vi "Deposition System Automation.vi"() -> ()   [LabVIEW 2018]
uses:
  <vilib>/MakerHub/LINX/Public/Peripherals/Digital/Digital Write 1 Chan.vi
  <vilib>/MakerHub/LINX/Public/Peripherals/Digital/Digital Write N Chans.vi
  <vilib>/MakerHub/LINX/Private/Local IO/LinxDigitalWrite.vi
  <vilib>/MakerHub/LINX/Public/Utilities/Check Channel.vi
  <vilib>/MakerHub/LINX/Public/Utilities/Open Serial.vi
  <vilib>/MakerHub/LINX/Private/Utilties/Generate Error.vi
  <vilib>/MakerHub/LINX/LMH-LINX.lvlib
panel:
  in  "Crashed?":bool
  in  "Arduino COM":refnum<visa-resource-name>="N/A"
  out "Turn On Turbo Pump":bool
  in  "Shut Down":bool
  in  "Turbo Pump":bool
  out "Turn On Pressure Gauge":bool
  in  "Rough Pump":bool
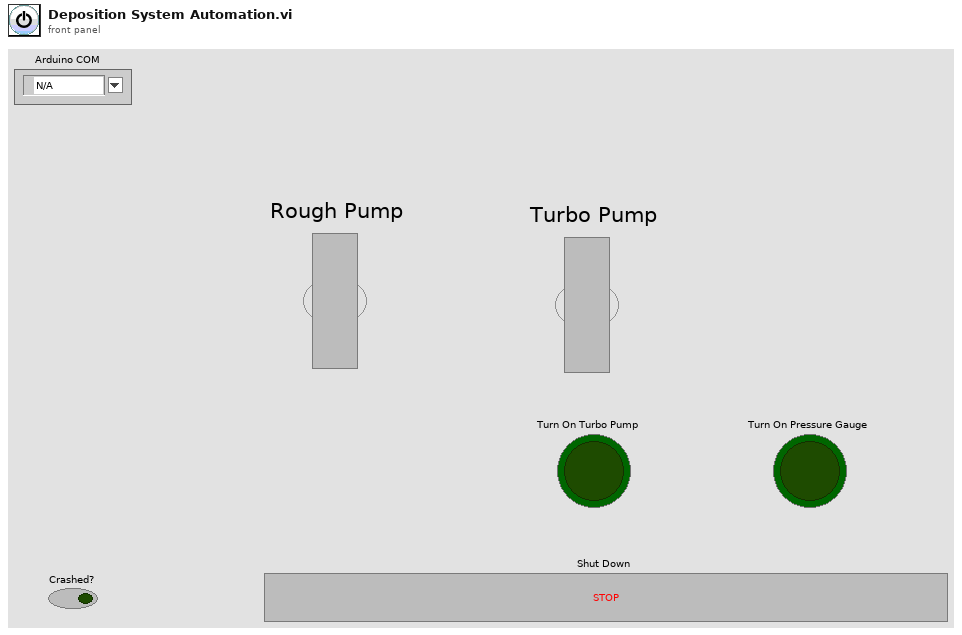
[diagram p1: front panel]
types:
  T1 = typedef "LMH-LINX.lvlib/LINX Ref.ctl" = cluster{"IO":T2, "Interface":T3, "LINX Device Config":T4}
  T2 = typedef "LMH-LINX.lvlib/Platform.ctl" = enum16{"Remote", "Local"}
  T3 = typedef "LMH-LINX.lvlib/Interface.ctl" = enum16{"Serial", "TCP"}
  T4 = typedef "LMH-LINX.lvlib/Device.lvlib/LINX Device Config.ctl" = cluster{"Interface":T3, "COM Port":refnum<visa-resource-name>, "TCP Configuration":T5, "Device Family":u8, "Device ID":u8, "Device Name":string, "TCP Ref":refnum<k5>, "Channels":T6}
  T5 = typedef "LMH-LINX.lvlib/Device.lvlib/TCP Config.ctl" = cluster{"IP Address":string, "Port":u16}
  T6 = typedef "LMH-LINX.lvlib/Channels.ctl" = cluster{"DI":u8[], "DO":u8[], "AI":u8[], "AO":u8[], "PWM":u8[], "QE":u8[], "UART":u8[], "I2C 2":u8[], "SPI":u8[], "CAN":u8[], "Servo":u8[], "AI Ref (V)":dbl, "AI Resolution (Bits)":u8, "AO Ref (V)":dbl, "AO Resolution (Bits)":u8}
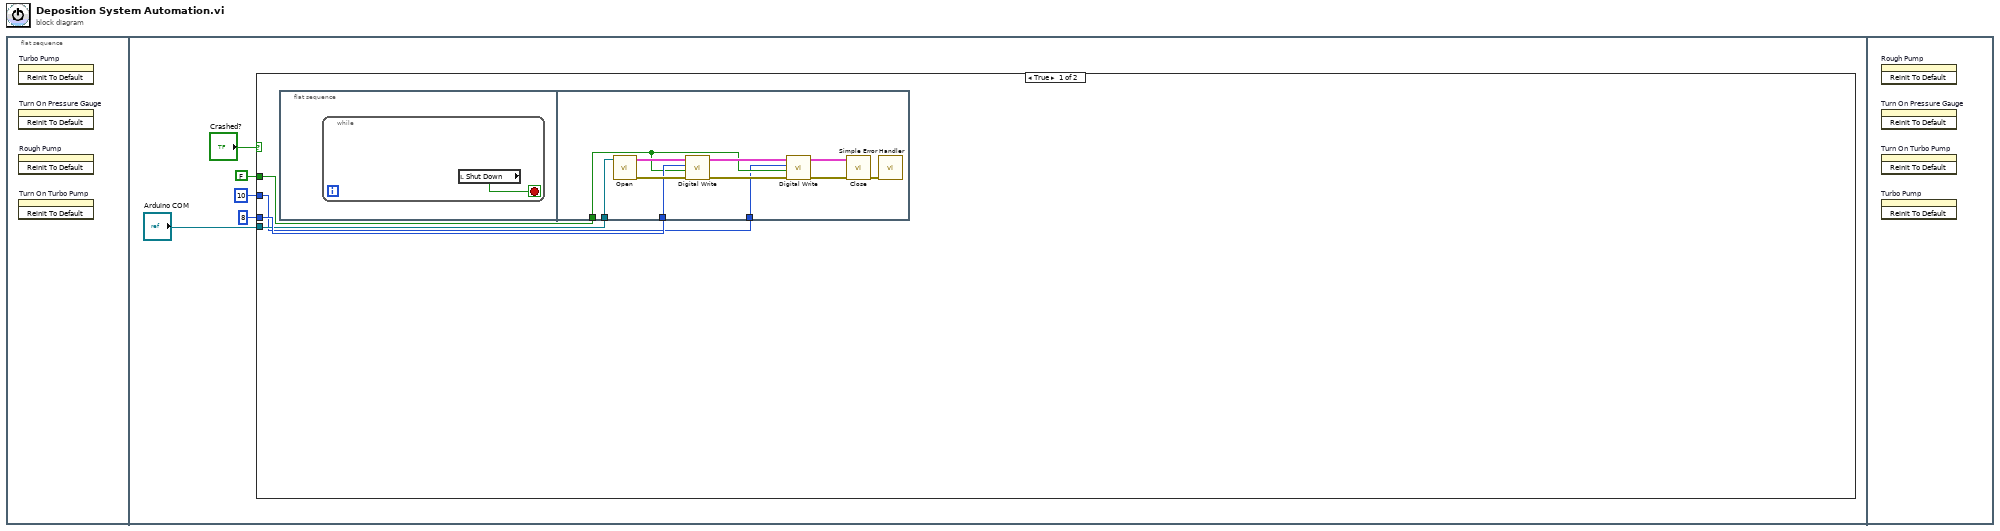
[diagram p0: block diagram]
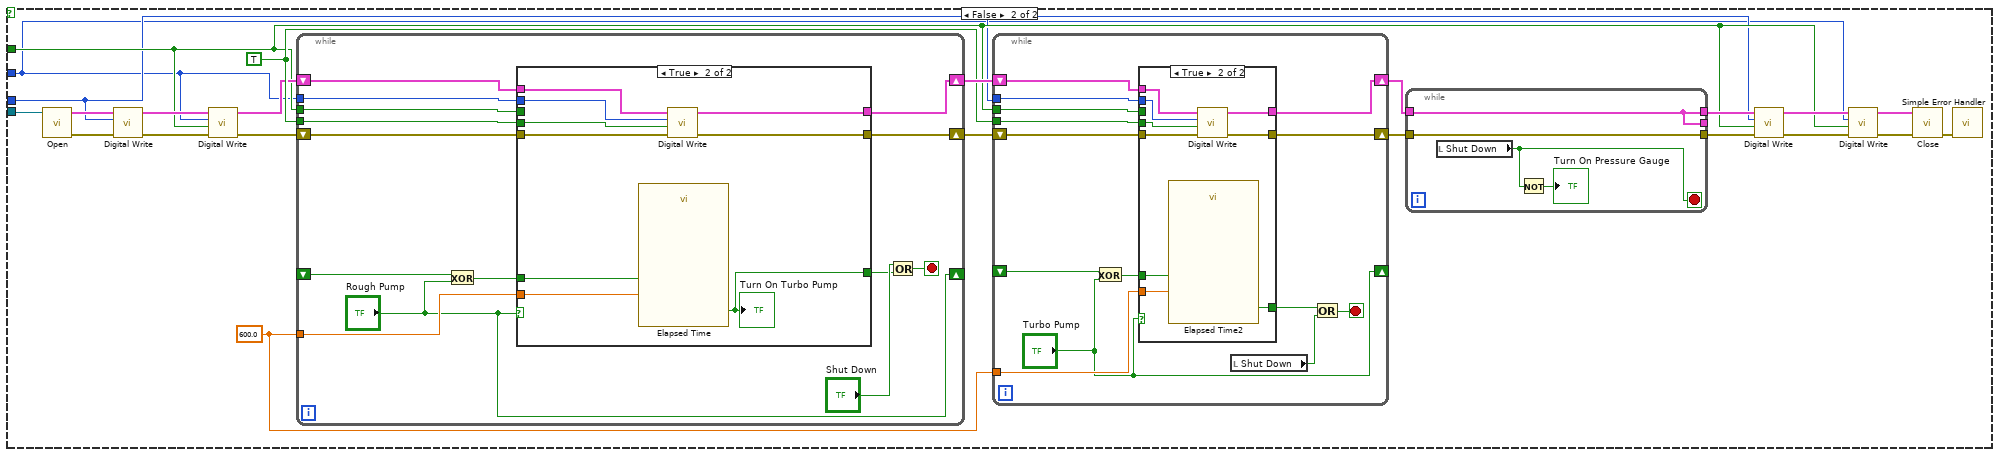
[diagram p2: hidden frame]
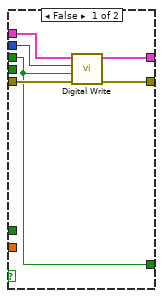
[diagram p3: hidden frame]
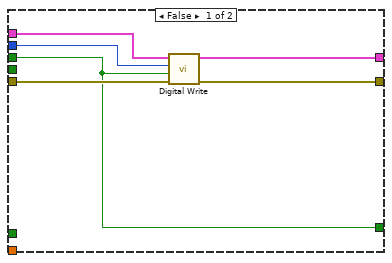
[diagram p4: hidden frame]
diagram:
  n1 = flat-sequence {
    frame #0 {
      n2 = invoke on="Turbo Pump" class="Bool (strict)" method="Reinit To Default"() -> ()  [unwired: 3 in, 3 out]
      n3 = invoke on="Turn On Pressure Gauge" class="Bool (strict)" method="Reinit To Default"() -> ()  [unwired: 3 in, 3 out]
      n4 = invoke on="Rough Pump" class="Bool (strict)" method="Reinit To Default"() -> ()  [unwired: 3 in, 3 out]
      n5 = invoke on="Turn On Turbo Pump" class="Bool (strict)" method="Reinit To Default"() -> ()  [unwired: 3 in, 3 out]
    }
    frame #1 {
      n6 = case shown="True" "Crashed?" {
        tunnel: u8 10 ("DO Channel") -> [w6 w22]
        tunnel: "Arduino COM" -> [w7 w36]
        tunnel: FALSE ("Time has Elapsed") -> [w9 w24]
        tunnel: u8 8 ("DO Channel") -> [w8 w23]
        frame True {
          n7 = flat-sequence {
            tunnel: w9 -> [w12]
            tunnel: w8 -> [w17]
            tunnel: w7 -> [w13]
            tunnel: w6 -> [w11]
            frame #0 {
              n8 = while {
                stop <- w10 stop-if-true
                n9 = local read "Shut Down"() -> (w10:bool)
              }
            }
            frame #1 {
              n10 = call-poly <vilib>:"Open.vi"("Serial Port"=w13) -> ("Error Out"=w19:errorcluster, "LINX Resource"=w18:T1)  [unwired: 8 in, 1 out]
              n11 = call-poly <vilib>:"Digital Write.vi"("Error In"=w19, "Output Value"=w12, "DO Channel"=w17, "LINX Resource"=w18) -> ("Error Out"=w21:errorcluster, "LINX Resource"=w20:T1)  [unwired: 6 in]
              n12 = call-poly <vilib>:"Digital Write.vi"("Error In"=w21, "Output Value"=w12, "DO Channel"=w11, "LINX Resource"=w20) -> ("Error Out"=w14:errorcluster, "LINX Resource"=w15:T1)  [unwired: 6 in]
              n13 = call <vilib>:"Close.vi"("Error In"=w14, "LINX Resource"=w15) -> ("Error Out"=w16:errorcluster)  [unwired: 9 in]
              n14 = call <vilib>:"Simple Error Handler.vi"("error in (no error)"=w16) -> ()  [unwired: 4 in, 5 out]
            }
          }
        }
        frame False {
          w41 = TRUE ("Output Value")
          w42 = 600.0 ("Time Target (s)")
          n15 = call-poly <vilib>:"Open.vi"("Serial Port"=w36) -> ("Error Out"=w35:errorcluster, "LINX Resource"=w34:T1)  [unwired: 8 in, 1 out]
          n16 = call-poly <vilib>:"Digital Write.vi"("Error In"=w35, "DO Channel"=w23, "LINX Resource"=w34) -> ("Error Out"=w40:errorcluster, "LINX Resource"=w39:T1)  [unwired: 7 in]
          n17 = call-poly <vilib>:"Digital Write.vi"("Error In"=w40, "Output Value"=w24, "DO Channel"=w22, "LINX Resource"=w39) -> ("Error Out"=w37:errorcluster, "LINX Resource"=w38:T1)  [unwired: 6 in]
          n18 = while {
            shift-right: [w89] -> w44
            shift-left: w38 -> [w91]
            shift-right: [w88] -> w43
            shift-left: w37 -> [w90]
            tunnel: w42 -> [w87]
            tunnel: w41 -> [w84]
            shift-right: ["Rough Pump"] -> _
            shift-left: _ -> [w82]
            tunnel: w22 -> [w79]
            tunnel: w24 -> [w78]
            stop <- w86 stop-if-true
            n19 = Exclusive Or(1:"Rough Pump", 2:w82) -> (0:w80:bool)
            n20 = case shown="True" "Rough Pump" {
              tunnel: w91 -> [w96 w106]
              tunnel: w90 -> [w95 w105]
              tunnel: w79 -> [w97 w104]
              tunnel: [w94 w103] -> w89
              tunnel: [w93 w102] -> w88
              tunnel: w87 -> [_ w101]
              tunnel: w84 -> [_ w100]
              tunnel: w78 -> [w92 _]
              tunnel: [w92 w99] -> w83
              tunnel: w80 -> [_ w98]
              frame False {
                n21 = call-poly <vilib>:"Digital Write.vi"("Error In"=w95, "Output Value"=w92, "DO Channel"=w97, "LINX Resource"=w96) -> ("Error Out"=w93:errorcluster, "LINX Resource"=w94:T1)  [unwired: 6 in]
              }
              frame True {
                n22 = call "Elapsed Time"("Time Target (s)"=w101, "Reset"=w98) -> ("Time has Elapsed"=w99:bool)  [unwired: 10 in, 7 out]
                "Turn On Turbo Pump" <- w99
                n23 = call-poly <vilib>:"Digital Write.vi"("Error In"=w105, "Output Value"=w100, "DO Channel"=w104, "LINX Resource"=w106) -> ("Error Out"=w102:errorcluster, "LINX Resource"=w103:T1)  [unwired: 6 in]
              }
            }
            n24 = Or(x="Shut Down", y=w83) -> (x .or. y?=w86:bool)
          }
          n25 = while {
            tunnel: w42 -> [w58]
            shift-right: [w62] -> w33
            shift-left: w44 -> [w60]
            shift-right: [w61] -> w32
            shift-left: w43 -> [w59]
            tunnel: w41 -> [w56]
            shift-right: ["Turbo Pump"] -> _
            shift-left: _ -> [w53]
            tunnel: w23 -> [w50]
            tunnel: w24 -> [w49]
            stop <- w54 stop-if-true
            n26 = Exclusive Or(1:"Turbo Pump", 2:w53) -> (0:w51:bool)
            n27 = case shown="True" "Turbo Pump" {
              tunnel: w50 -> [w64 w77]
              tunnel: [w66 w76] -> w62
              tunnel: [w65 w75] -> w61
              tunnel: w60 -> [w68 w74]
              tunnel: w59 -> [w67 w73]
              tunnel: w58 -> [_ w72]
              tunnel: w56 -> [_ w71]
              tunnel: w49 -> [w63 _]
              tunnel: [w63 w70] -> w55
              tunnel: w51 -> [_ w69]
              frame False {
                n28 = call-poly <vilib>:"Digital Write.vi"("Error In"=w67, "Output Value"=w63, "DO Channel"=w64, "LINX Resource"=w68) -> ("Error Out"=w65:errorcluster, "LINX Resource"=w66:T1)  [unwired: 6 in]
              }
              frame True {
                n29 = call "Elapsed Time2"("Time Target (s)"=w72, "Reset"=w69) -> ("Time has Elapsed"=w70:bool)  [unwired: 10 in, 7 out]
                n30 = call-poly <vilib>:"Digital Write.vi"("Error In"=w73, "Output Value"=w71, "DO Channel"=w77, "LINX Resource"=w74) -> ("Error Out"=w75:errorcluster, "LINX Resource"=w76:T1)  [unwired: 6 in]
              }
            }
            n31 = local read "Shut Down"() -> (w57:bool)
            n32 = Or(x=w55, y=w57) -> (x .or. y?=w54:bool)
          }
          n33 = while {
            tunnel: [w48] -> _
            tunnel: w33 -> [w48]
            tunnel: [w48] -> w25
            tunnel: [w47] -> w26
            tunnel: w32 -> [w47]
            stop <- w45 stop-if-true
            n34 = local read "Shut Down"() -> (w45:bool)
            n35 = Not(x=w45) -> (.not. x?=→"Turn On Pressure Gauge":bool)
          }
          n36 = call-poly <vilib>:"Digital Write.vi"("Error In"=w26, "Output Value"=w24, "DO Channel"=w23, "LINX Resource"=w25) -> ("Error Out"=w29:errorcluster, "LINX Resource"=w28:T1)  [unwired: 6 in]
          n37 = call-poly <vilib>:"Digital Write.vi"("Error In"=w29, "Output Value"=w24, "DO Channel"=w22, "LINX Resource"=w28) -> ("Error Out"=w31:errorcluster, "LINX Resource"=w30:T1)  [unwired: 6 in]
          n38 = call <vilib>:"Close.vi"("Error In"=w31, "LINX Resource"=w30) -> ("Error Out"=w27:errorcluster)  [unwired: 9 in]
          n39 = call <vilib>:"Simple Error Handler.vi"("error in (no error)"=w27) -> ()  [unwired: 4 in, 5 out]
        }
      }
    }
    frame #2 {
      n40 = invoke on="Rough Pump" class="Bool (strict)" method="Reinit To Default"() -> ()  [unwired: 3 in, 3 out]
      n41 = invoke on="Turn On Pressure Gauge" class="Bool (strict)" method="Reinit To Default"() -> ()  [unwired: 3 in, 3 out]
      n42 = invoke on="Turn On Turbo Pump" class="Bool (strict)" method="Reinit To Default"() -> ()  [unwired: 3 in, 3 out]
      n43 = invoke on="Turbo Pump" class="Bool (strict)" method="Reinit To Default"() -> ()  [unwired: 3 in, 3 out]
    }
  }
